vi "add.vi"(10 "b":dbl, 11 "a":dbl) -> (3 "sum":dbl)   [LabVIEW 2023]
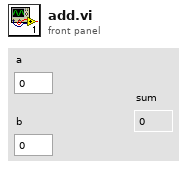
[diagram p1: front panel]
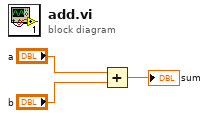
[diagram p0: block diagram]
diagram:
  n1 = Add(x="a", y="b") -> (x+y=→"sum":dbl)
